vi "__Safely Recursive File List.vi"(6 "pattern":string, 8 "error in (no error)":errorcluster, 10 "Treat LLBs as Folders?":bool, 11 "Path":path) -> (0 "error out":errorcluster, 2 "All Files in Dir":path[](array[path]), 3 "dup Folder Path":path)   [LabVIEW 2019, in "LabVIEW-ProviderShell.lvlib"]
uses:
  LabVIEW-ProviderShell.lvlib
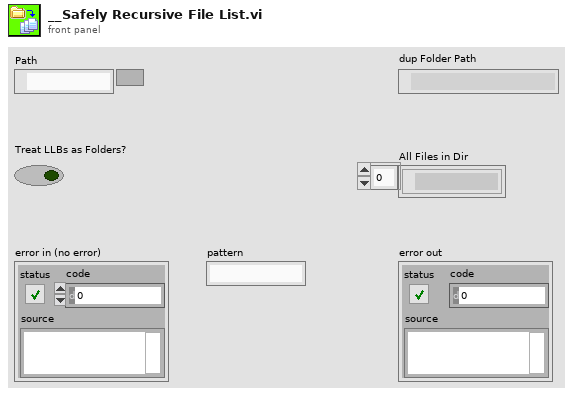
[diagram p1: front panel]
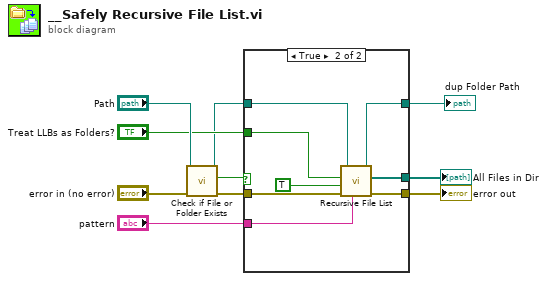
[diagram p0: block diagram]
diagram:
  n1 = call <vilib>:"Check if File or Folder Exists.vi"("error in (no error)"="error in (no error)", "path"="Path") -> ("error out"=w3:errorcluster, "file or folder exists?"=w2:bool, "dup path"=w5:path)  [unwired: 7 in]
  n2 = case shown="True" w2 {
    tunnel: [w12 w20] -> w10
    tunnel: [_ w19] -> w9
    tunnel: "pattern" -> [_ w17]
    tunnel: "Treat LLBs as Folders?" -> [_ w16]
    tunnel: w5 -> [w11 w15]
    tunnel: w3 -> [w12 w14]
    tunnel: [w11 w13] -> w1
    frame False {
    }
    frame True {
      n3 = call <vilib>:"Recursive File List.vi"("pattern"=w17, "error in (no error)"=w14, "Continue Recursing on Error? (F)"=TRUE ("Continue Recursing on Error?"), "Treat LLBs as Folders?"=w16, "Folder Path"=w15) -> ("error out"=w20:errorcluster, "All Files in Dir"=w19:path[], "dup Folder Path"=w13:path)  [unwired: 2 in, 2 out]
    }
  }
  "error out" <- w10
  "All Files in Dir" <- w9
  "dup Folder Path" <- w1
